vi "DSP_GetFftOutRealFloatScale.vi"(0 "Board Handle":u64, 1 "error in (no error)":errorcluster) -> (2 "Board Handle Out":u64, 3 "Value":sgl, 4 "error out":errorcluster)   [LabVIEW 2009]
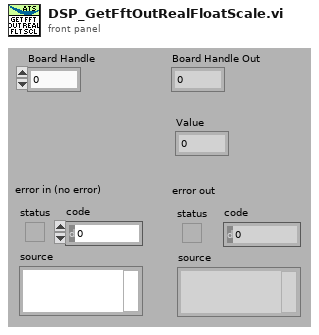
[diagram p1: front panel]
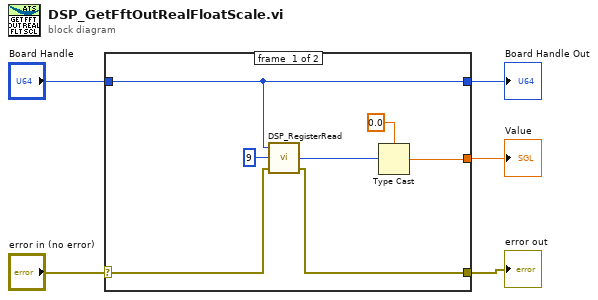
[diagram p0: block diagram]
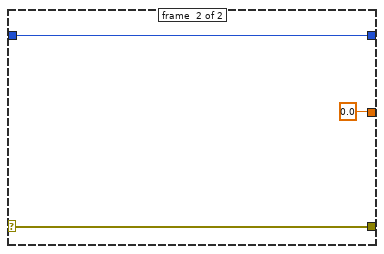
[diagram p2: hidden frame]
diagram:
  n1 = case shown="No Error" "error in (no error)" {
    selector: "error in (no error)" -> [w11 w15]
    tunnel: [w10 w15] -> w4
    tunnel: [w12 w14] -> w3
    tunnel: "Board Handle" -> [w12 w14]
    tunnel: [w6 sgl 0.0] -> w1
    frame #0 {
      n2 = call "DSP_RegisterRead.vi"("error in (no error)"=w11, "Offset"=u32 9, "Board Handle"=w12) -> ("error out"=w10:errorcluster, "Value"=w8:u32)  [unwired: 1 out]
      n3 = Type Cast(type=sgl 0.0, x=w8) -> (*(type *) &x=w6:sgl)
    }
    frame #1 {
    }
  }
  "Board Handle Out" <- w3
  "error out" <- w4
  "Value" <- w1
